vi "Circuit Protection.vi"(0 "VISA Resource Name":refnum<visa-resource-name>, 11 "error in (no error)":errorcluster {"code" format="%.0x"}) -> (4 "VISA Resource Name Out":refnum<visa-resource-name>, 15 "error out":errorcluster {"code" format="%.0x"})   [LabVIEW 2014, in "Agilent ESG Series.lvlib"]
doc: "This VI checks to see if the signal generator's reverse power protection circutry has been activated and resets it if it has."
uses:
  Agilent ESG Series.lvlib
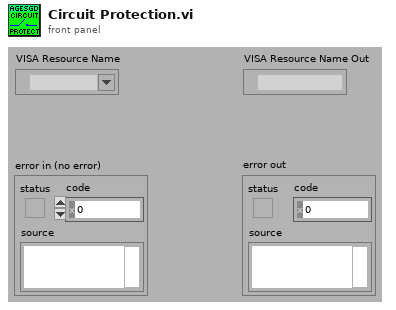
[diagram p1: front panel]
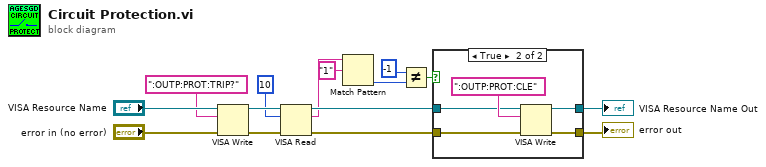
[diagram p0: block diagram]
diagram:
  n1 = VISA Write(VISA resource name="VISA Resource Name", write buffer=":OUTP:PROT:TRIP?" ("write buffer (\"\")"), error in (no error)="error in (no error)") -> (VISA resource name out=w13:refnum<visa-resource-name>, error out=w12:errorcluster)  [unwired: 1 out]
  n2 = VISA Read(VISA resource name=w13, byte count=u32 10 ("byte count (0)"), error in (no error)=w12) -> (VISA resource name out=w10:refnum<visa-resource-name>, read buffer=w2:string, error out=w11:errorcluster)  [unwired: 1 out]
  n3 = Match Pattern(string=w2, regular expression="1") -> (offset past match=w5:i32)  [unwired: 1 in, 3 out]
  n4 = Not Equal?(x=-1, y=w5) -> (x != y?=w3:bool)
  n5 = case shown="True" w3 {
    tunnel: [w16 w21] -> w8
    tunnel: [w17 w20] -> w9
    tunnel: w10 -> [w17 w19]
    tunnel: w11 -> [w16 w18]
    frame False {
    }
    frame True {
      n6 = VISA Write(VISA resource name=w19, write buffer=":OUTP:PROT:CLE", error in (no error)=w18) -> (VISA resource name out=w20:refnum<visa-resource-name>, error out=w21:errorcluster)  [unwired: 1 out]
    }
  }
  "error out" <- w8
  "VISA Resource Name Out" <- w9
